vi "FTW-Test-Actor-Stress.vi"() -> (0 "Test Result":errorcluster)   [LabVIEW 2014]
uses:
  src/core/error/FTW-ERR-Assert-DeveloperError.vi
  src/core/error/FTW-ERR-ThrowError.vi
  src/core/error/FTW-ERR-NoErrorConstant.vi
  src/core/error/FTW-ERR-CallChain.vi
  src/core/string/FTW-STR-ReplaceWhitespace.vi
  src/core/actor/connector/FTW-Actor-Connector.lvclass
panel:
  out "Actor Pool Spawn":dbl format="Actor Pool Spawn: %_3psec"
  out "Total Elapsed Time":dbl format="Messaging Time: %_3psec"
  out "\"FTW: Ping\" Times":cluster{dbl[]}[](graph)
  in  "Test to Perform":T1(radio)=enum."Parallel: 10x10"
  out "\"PING\" Times":cluster{dbl[]}[](graph)
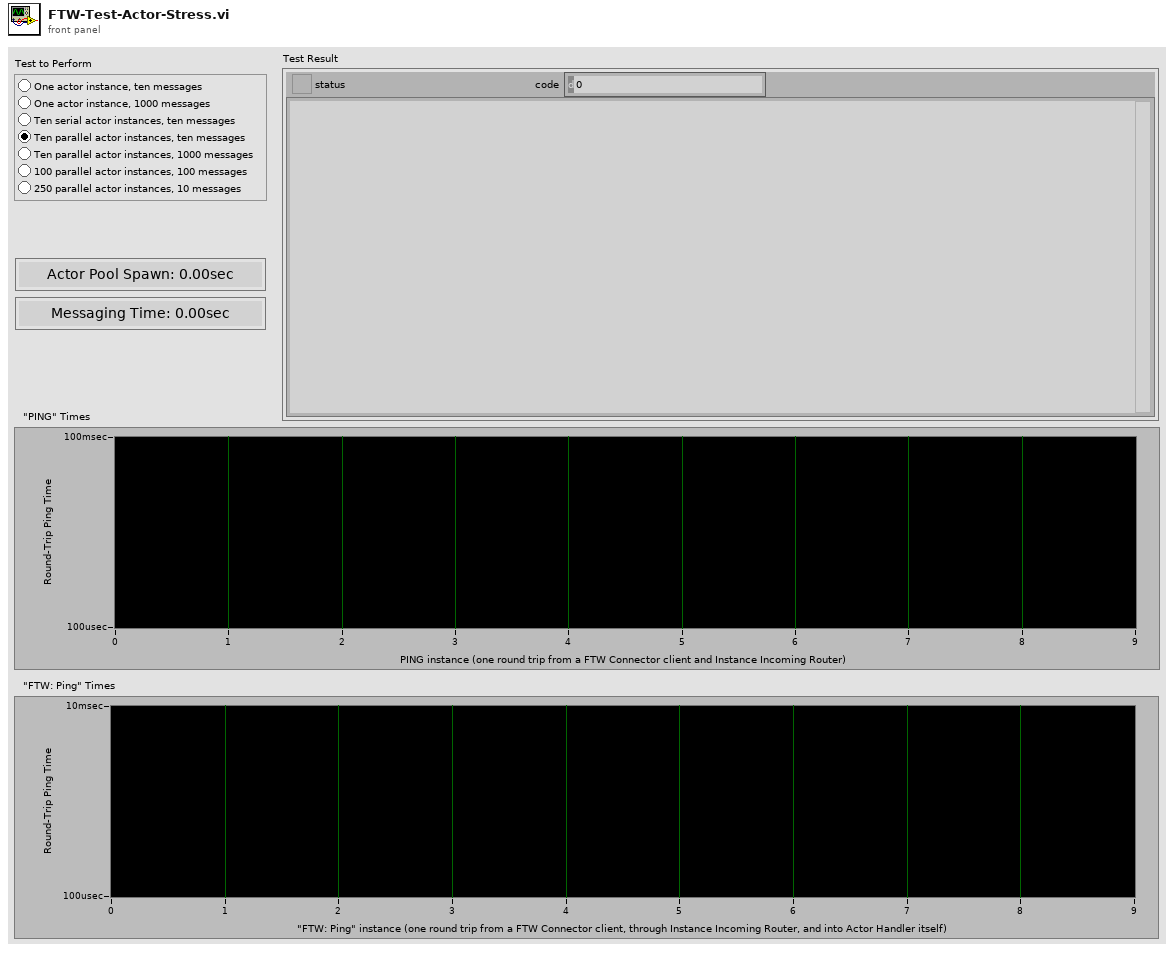
[diagram p1: front panel]
types:
  T1 = enum32{"Serial: 1x10", "Serial: 1x1000", "Serial: 10x10", "Parallel: 10x10", "Parallel: 10x100", "Parallel: 100x100", "Parallel: 250x10"}
  T2 = cluster{i32, "Initial Handshake Response":string, "Instance Inbox Address":string, "error out":errorcluster}
  T3 = cluster{i32, bool, bool, "Timed out?":bool, "error out":errorcluster, dbl[], dbl[]}
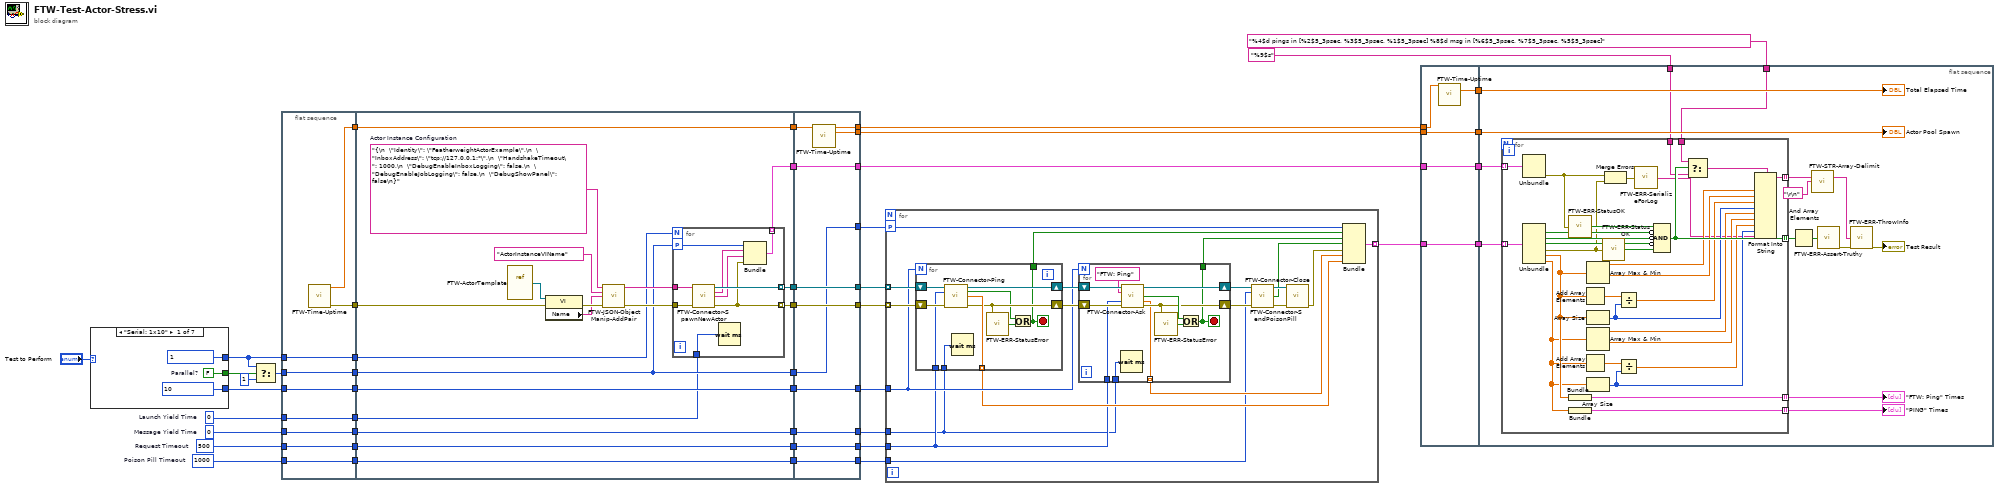
[diagram p0: block diagram]
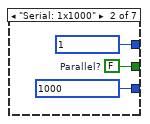
[diagram p2: hidden frame]
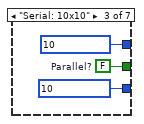
[diagram p3: hidden frame]
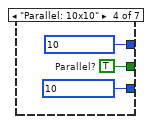
[diagram p4: hidden frame]
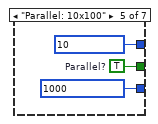
[diagram p5: hidden frame]
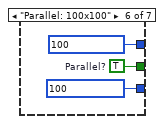
[diagram p6: hidden frame]
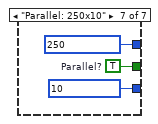
[diagram p7: hidden frame]
diagram:
  w4 = u32 0  # Message Yield Time
  w8 = u32 0  # Launch Yield Time
  w10 = 1000  # Poison Pill Timeout
  w12 = 500  # Request Timeout
  n1 = case shown="\"Serial: 1x10\"" "Test to Perform" {
    tunnel: [1 1 10 10 10 100 250] -> w16
    tunnel: [10 1000 10 10 1000 100 10] -> w14
    tunnel: [w46 w49 w52 w55 w58 w61 w64] -> w20
    frame "Serial: 1x10" {
      w46 = FALSE  # Parallel?
    }
    frame "Serial: 1x1000" {
      w49 = FALSE  # Parallel?
    }
    frame "Serial: 10x10" {
      w52 = FALSE  # Parallel?
    }
    frame "Parallel: 10x10" {
      w55 = TRUE  # Parallel?
    }
    frame "Parallel: 10x100" {
      w58 = TRUE  # Parallel?
    }
    frame "Parallel: 100x100" {
      w61 = TRUE  # Parallel?
    }
    frame "Parallel: 250x10" {
      w64 = TRUE  # Parallel?
    }
  }
  n2 = Select(t=w16, s=w20, f=1) -> (s? t:f=w18:i32)
  n3 = flat-sequence {
    tunnel: [w75] -> w24
    tunnel: [w71] -> w23
    tunnel: [w74] -> w19
    tunnel: w18 -> [w74]
    tunnel: [w73] -> w17
    tunnel: w16 -> [w73]
    tunnel: [w72] -> w15
    tunnel: w14 -> [w72]
    tunnel: [w70] -> w13
    tunnel: w12 -> [w70]
    tunnel: [w69] -> w11
    tunnel: w10 -> [w69]
    tunnel: [w68] -> w9
    tunnel: w8 -> [w68]
    tunnel: [w67] -> w5
    tunnel: w4 -> [w67]
    tunnel: [w88] -> w36
    tunnel: [w87] -> w35
    tunnel: [w80] -> w34
    tunnel: [w82] -> w33
    tunnel: [w86] -> w32
    tunnel: [w84] -> w31
    tunnel: [w79] -> w27
    tunnel: [w78] -> w25
    tunnel: w24 -> [w85]
    tunnel: w23 -> [w84]
    tunnel: w19 -> [w82]
    tunnel: w17 -> [w81]
    tunnel: w15 -> [w80]
    tunnel: w13 -> [w79]
    tunnel: w11 -> [w78]
    tunnel: w9 -> [w77]
    tunnel: [w76] -> w6
    tunnel: w5 -> [w76]
    tunnel: [w110] -> w41
    tunnel: [w111] -> w42
    tunnel: [w112] -> w43
    tunnel: [w113] -> w44
    tunnel: [w114] -> w45
    tunnel: w36 -> [w114]
    tunnel: w35 -> [w113]
    tunnel: w34 -> [w112]
    tunnel: w33 -> [w111]
    tunnel: w32 -> [w110]
    tunnel: w31 -> [w109]
    tunnel: [w108] -> w29
    tunnel: [w107] -> w28
    tunnel: w27 -> [w107]
    tunnel: [w106] -> w26
    tunnel: w25 -> [w106]
    tunnel: [w105] -> w3
    tunnel: [w104] -> w7
    tunnel: w6 -> [w104]
    frame #0 {
      n4 = call "FTW-Time-Uptime.vi"() -> ("Current Uptime"=w71:dbl, "error out"=w75:errorcluster)  [unwired: 13 in, 1 out]
    }
    frame #1 {
      w93 = "{\n  \"Identity\": \"FeatherweightActorExample\",\n  \"InboxAddress\": \"tcp://127.0.0.1:*\",\n  \"HandshakeTimeout\": 1000,\n  \"DebugEnableInboxLogging\": false,\n  \"DebugEnableJobLogging\": false,\n  \"DebugShowPanel\": false\n}"  # Actor Instance Configuration
      n5 = vi-ref "FTW-ActorTemplate.vi"() -> (w94:refnum<vi>)
      n6 = property class="VI"(reference=w94, error in=w85) -> (error out=w91:errorcluster, "Name"=w83:string)  [unwired: 1 out]
      n7 = call "FTW-JSON-ObjectManip-AddPair.vi"("Input JSON Object"=w93, "Key"="ActorInstanceVIName", "Value"=w83, "error in"=w91) -> ("Output JSON Object"=w92:string, "error out"=w90:errorcluster)  [unwired: 10 in]
      n8 = for {
        N: w81 -> [_]
        tunnel: w92 -> [w96]
        tunnel: w90 -> [w103]
        tunnel: [w102] -> w88 mode=indexing
        tunnel: [w98] -> w87 mode=indexing
        tunnel: [w99] -> w86 mode=indexing
        workers-P: w82 -> [w97]
        tunnel: w77 -> [w95]
        n9 = call "FTW-Connector-SpawnNewActor.vi"("Instance Configuration"=w96, "error in"=w103) -> ("FTW Actor Connector"=w102:refnum<class "FTW-Actor-Connector.lvclass">, "Initial Handshake Response"=w101:string, "Instance Inbox Address"=w100:string, "error out"=w98:errorcluster)  [unwired: 10 in]
        n10 = Wait (ms)(milliseconds to wait=w95) -> ()  [unwired: 1 out]
        n11 = Bundle(w97, "Initial Handshake Response"=w101, "Instance Inbox Address"=w100, "error out"=w98) -> (w99:T2)  [unwired: 1 in]
      }
    }
    frame #2 {
      n12 = call "FTW-Time-Uptime.vi"("Previous Uptime"=w109) -> ("Current Uptime"=w105:dbl, "Elapsed Time"=w108:dbl)  [unwired: 12 in, 1 out]
    }
  }
  n13 = for {
    tunnel: w45 -> [w132] mode=indexing
    tunnel: w44 -> [w131] mode=indexing
    tunnel: w43 -> [w126]
    workers-P: w42 -> [w125]
    tunnel: [w122] -> w40 mode=indexing
    tunnel: w28 -> [w117]
    tunnel: w26 -> [w116]
    tunnel: w7 -> [w115]
    n14 = for {
      N: w126 -> [_]
      tunnel: [w141] -> w118 mode=indexing
      shift-right: [w142] -> w130
      shift-left: w132 -> [w144]
      shift-right: [w140] -> w129
      shift-left: w131 -> [w143]
      tunnel: [w137] -> w124
      tunnel: w117 -> [w136]
      tunnel: w115 -> [w135]
      stop <- w137 stop-if-true
      n15 = call-dynamic "FTW-Connector-Ping.vi"("FTW Actor Connector Type"=w144, "Timeout"=w136, "error in"=w143) -> ("FTW Actor Connector"=w142:refnum<class "FTW-Actor-Connector.lvclass">, "Timed out?"=w138:bool, "Roundtrip Time"=w141:dbl, "error out"=w140:errorcluster)  [unwired: 9 in]
      n16 = Wait (ms)(milliseconds to wait=w135) -> ()  [unwired: 1 out]
      n17 = call "FTW-ERR-StatusError.vi"("error to check"=w140) -> ("Error?"=w139:bool)
      n18 = Or(x=w138, y=w139) -> (x .or. y?=w137:bool)
    }
    n19 = for {
      N: w126 -> [_]
      tunnel: [w150] -> w119 mode=indexing
      shift-right: [w153] -> w128
      shift-left: w130 -> [w154]
      shift-right: [w151] -> w127
      shift-left: w129 -> [w149]
      tunnel: [w148] -> w123
      tunnel: w117 -> [w147]
      tunnel: w115 -> [w146]
      stop <- w148 stop-if-true
      n20 = Wait (ms)(milliseconds to wait=w146) -> ()  [unwired: 1 out]
      n21 = call "FTW-Connector-Ask.vi"("FTW Actor Connector"=w154, "Request Header"="FTW: Ping", "Timeout"=w147, "error in"=w149) -> ("FTW Actor Connector out"=w153:refnum<class "FTW-Actor-Connector.lvclass">, "Timed out?"=w152:bool, "Roundtrip Time"=w150:dbl, "error out"=w151:errorcluster)  [unwired: 7 in, 1 out]
      n22 = call "FTW-ERR-StatusError.vi"("error to check"=w151) -> ("Error?"=w155:bool)
      n23 = Or(x=w152, y=w155) -> (x .or. y?=w148:bool)
    }
    n24 = call-dynamic "FTW-Connector-SendPoisonPill.vi"("FTW Actor Connector"=w128, "Timeout"=w116, "error in"=w127) -> ("FTW Actor Connector out"=w134:refnum<class "FTW-Actor-Connector.lvclass">, "Timed out?"=w121:bool, "error out"=w133:errorcluster)  [unwired: 9 in, 1 out]
    n25 = call-dynamic "FTW-Connector-Close.vi"("FTW Actor Connector"=w134, "error in"=w133) -> ("error out"=w120:errorcluster)  [unwired: 13 in]
    n26 = Bundle(w125, w124, w123, "Timed out?"=w121, "error out"=w120, w119, w118) -> (w122:T3)  [unwired: 1 in]
  }
  n27 = flat-sequence {
    tunnel: w40 -> [w159]
    tunnel: w41 -> [w160]
    tunnel: [w160] -> w39
    tunnel: [w159] -> w38
    tunnel: [w158] -> w37
    tunnel: [w157] -> w30
    tunnel: w29 -> [w157]
    tunnel: w3 -> [w156]
    tunnel: w39 -> [w175]
    tunnel: w38 -> [w174]
    tunnel: w37 -> [w172]
    tunnel: w30 -> [w170]
    tunnel: "%4$d pings in [%2$5_3psec, %3$5_3psec, %1$5_3psec] %8$d msg in [%6$5_3psec, %7$5_3psec, %5$5_3psec]" ("format string") -> [w166]
    tunnel: "%9$s" ("format string") -> [w161]
    frame #0 {
      n28 = call "FTW-Time-Uptime.vi"("Previous Uptime"=w156) -> ("Elapsed Time"=w158:dbl)  [unwired: 12 in, 2 out]
    }
    frame #1 {
      n29 = for {
        tunnel: w175 -> [w205] mode=indexing
        tunnel: w174 -> [w204] mode=indexing
        tunnel: w166 -> [w179]
        tunnel: [w193] -> w173 mode=indexing
        tunnel: [w195] -> w171 mode=indexing
        tunnel: [w198] -> w164 mode=indexing
        tunnel: [w194] -> w167 mode=indexing
        tunnel: w161 -> [w176]
        n30 = Unbundle(w205) -> ("error out"=w197:errorcluster)  [unwired: 3 out]
        n31 = Unbundle(w204) -> (w202:bool, w201:bool, "Timed out?"=w200:bool, "error out"=w192:errorcluster, w191:dbl[], w185:dbl[])  [unwired: 1 out]
        n32 = call "FTW-ERR-StatusOK.vi"("error to check"=w197) -> ("Status OK?"=w203:bool)
        n33 = Bundle(w191) -> (w194:cluster{dbl[]})  [unwired: 1 in]
        n34 = Bundle(w185) -> (w193:cluster{dbl[]})  [unwired: 1 in]
        n35 = Add Array Elements(numeric array=w191) -> (sum=w196:dbl)
        n36 = Add Array Elements(numeric array=w185) -> (sum=w186:dbl)
        n37 = Array Max & Min(array=w191) -> (max value=w190:dbl, min value=w189:dbl)  [unwired: 2 out]
        n38 = Array Size(array=w191) -> (size(s)=w187:i32)
        n39 = Array Max & Min(array=w185) -> (max value=w184:dbl, min value=w183:dbl)  [unwired: 2 out]
        n40 = Array Size(array=w185) -> (size(s)=w181:i32)
        n41 = call "FTW-ERR-StatusOK.vi"("error to check"=w192) -> ("Status OK?"=w199:bool)
        n42 = Merge Errors(w197, w192) -> (w180:errorcluster)
        n43 = Divide(x=w196, y=w187) -> (x/y=w188:dbl)
        n44 = Divide(x=w186, y=w181) -> (x/y=w182:dbl)
        n45 = call "FTW-ERR-SerializeForLog.vi"("error in"=w180) -> ("Serialized Error"=w177:string)
        n46 = Compound Arithmetic op=AND(w203, invert w202, invert w201, invert w200, w199) -> (w195:bool)
        n47 = Select(t=w179, s=w195, f=w176) -> (s? t:f=w178:string)
        n48 = Format Into String(format string=w178, w190, w189, w188, w187, w184, w183, w182, w181, w177) -> (resulting string=w198:string)  [unwired: 2 in, 1 out]
      }
      "\"PING\" Times" <- w173
      "\"FTW: Ping\" Times" <- w167
      n49 = And Array Elements(Boolean array=w171) -> (logical AND=w168:bool)
      n50 = call "FTW-STR-Array-Delimit.vi"("Array of Strings"=w164, "Delimiter"="\r\n") -> ("Delimited String"=w163:string)  [unwired: 13 in]
      n51 = call "FTW-ERR-Assert-Truthy.vi"("Expected Truthy"=w168) -> ("error out"=w169:errorcluster)  [unwired: 14 in]
      n52 = call "FTW-ERR-ThrowInfo.vi"("Informational Message"=w163, "error in"=w169) -> ("error out"=→"Test Result":errorcluster)  [unwired: 13 in]
      "Total Elapsed Time" <- w172
      "Actor Pool Spawn" <- w170
    }
  }
